vi "Update dp Jumo.vi"(8 "error in":errorcluster, 10 "dp Jumo":waveform(dbl)[](array[waveform]), 11 "DeepU Results in":refnum<class "DeepU Results.lvclass">) -> (0 "error out":errorcluster, 3 "DeepU Results out":refnum<class "DeepU Results.lvclass">)   [LabVIEW 2019, in "Results.lvlib" / "DeepU Results.lvclass"]
uses:
  DeepU Results.lvclass
  DeepU Results.lvclass/DeepU Results.ctl
  <vilib>/Analysis/NI_AALBase.lvlib
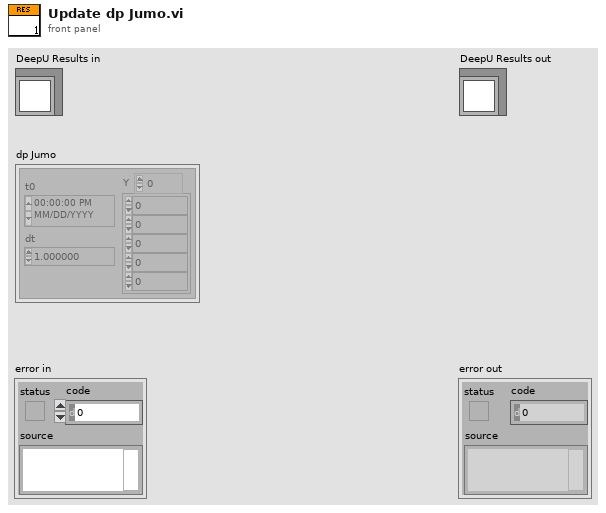
[diagram p1: front panel]
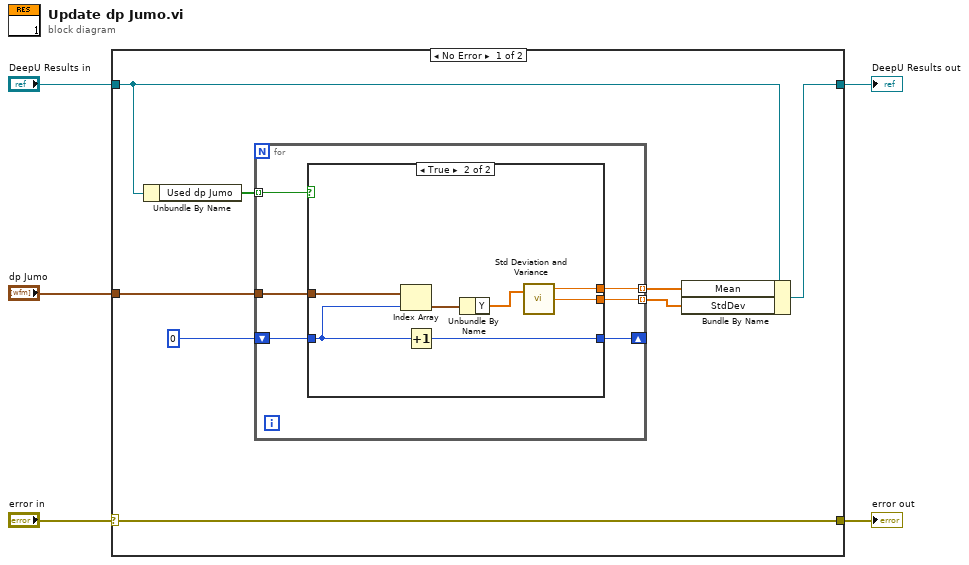
[diagram p0: block diagram]
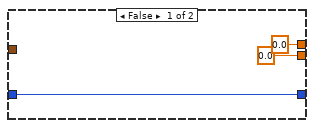
[diagram p2: hidden frame]
diagram:
  n1 = case shown="No Error" "error in" {
    selector: "error in" -> [w13 w30]
    tunnel: [w13 w30] -> w1
    tunnel: [w12 w31] -> w2
    tunnel: "DeepU Results in" -> [w11 w31]
    tunnel: "dp Jumo" -> [w10 _]
    frame No Error {
      n2 = Unbundle By Name(w11) -> ("Used dp Jumo"=w8:bool[])
      n3 = for {
        tunnel: w8 -> [w18] mode=indexing
        tunnel: w10 -> [w19]
        shift-right: [w16] -> _
        shift-left: 0 -> [w17]
        tunnel: [w15] -> w7 mode=indexing
        tunnel: [w14] -> w6 mode=indexing
        n4 = case shown="True" w18 {
          tunnel: w19 -> [_ w29]
          tunnel: w17 -> [w22 w28]
          tunnel: [w22 w27] -> w16
          tunnel: [0.0 ("mean") w24] -> w15
          tunnel: [0.0 ("standard deviation") w23] -> w14
          frame False {
          }
          frame True {
            n5 = Index Array(array=w29, index=w28) -> (element=w26:waveform(dbl))
            n6 = Increment(x=w28) -> (x+1=w27:i32)
            n7 = Unbundle By Name(w26) -> ("Y"=w25:dbl[])
            n8 = call <vilib>:"Std Deviation and Variance.vi"("X"=w25) -> ("mean"=w24:dbl, "standard deviation"=w23:dbl)  [unwired: 1 in, 1 out]
          }
        }
      }
      n9 = Bundle By Name(cluster=w11, "Mean"=w7, "StdDev"=w6) -> (w12:refnum<class "DeepU Results.lvclass">)
    }
    frame Error {
    }
  }
  "error out" <- w1
  "DeepU Results out" <- w2
